vi "Untitled 1.vi"   [LabVIEW 2024]
uses:
  <instrlib>/EFmeter/EFmeter.lvlib
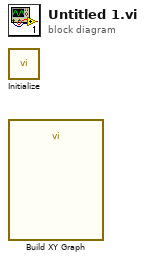
[diagram p0: block diagram]
diagram:
  n1 = call <instrlib>:"Initialize.vi"() -> ()  [unwired: 10 in, 2 out]
  n2 = call "Build XY Graph"() -> ("XY Graph"=w1:cluster{"X":dbl[], "Y":dbl[]}[])  [unwired: 10 in, 1 out]
